vi "Send Command.vi"(8 "error in (no error)":errorcluster, 10 "Command":u8(ring)=27 items=["Cancel"=24, "Clear"=25, "CSR"=28, "Echo"=27, "Filter"=15, "Gcal"=18, "Goto"=16, "Grtid?"=19, "Grtsel"=26, "NOVRAM Read"=56, "NOVRAM Write"=59, "Reset"=255, "Scan"=12, "Scan Up"=9, "Scan Down"=3, "Serial?"=33, "Slew Up"=8, "Slew Down"=2, "Slit Reset"=43, "Slit?"=30, "Sltadj"=14, "Speed"=13, "Speed?"=21, "Step Down"=1, "Step Up"=7, "S1adj"=31, "S2adj"=32, "S3adj"=34, "S1cal"=22, "S2cal"=23, "S3cal"=35, "Test"=17, "Type"=57, "Wave?"=29, "Zero"=52], 11 "VISA resource name":refnum<visa-resource-name>) -> (0 "error out":errorcluster, 2 "response":u8, 3 "VISA resource name out":refnum<visa-resource-name>)   [LabVIEW 2012, in "Digikrom DK24x.lvlib"]
doc: "Begins the communication sequence for the specified command."
uses:
  Digikrom DK24x.lvlib
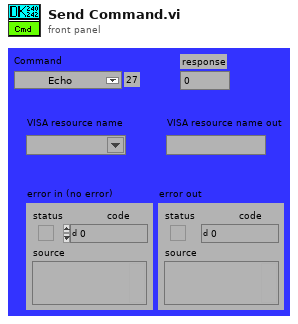
[diagram p1: front panel]
types:
  T1 = typedef "Semaphore RefNum" = refnum<k1>
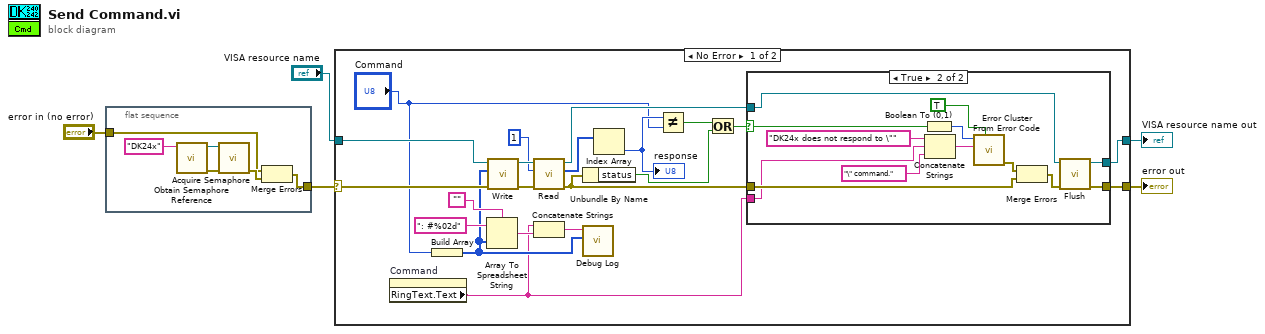
[diagram p0: block diagram]
diagram:
  n1 = flat-sequence {
    tunnel: "error in (no error)" -> [w7]
    tunnel: [w6] -> w1
    frame #0 {
      n2 = call <vilib>:"Obtain Semaphore Reference.vi"("name (unnamed)"="DK24x") -> ("error out"=w9:errorcluster, "semaphore"=w10:T1)  [unwired: 2 in, 3 out]
      n3 = call <vilib>:"Acquire Semaphore.vi"("error in (no error)"=w9, "semaphore"=w10) -> ("error out"=w8:errorcluster)  [unwired: 1 in, 4 out]
      n4 = Merge Errors(w7, w8) -> (w6:errorcluster)
    }
  }
  n5 = case shown="No Error" w1 {
    selector: w1 -> [w19 w48]
    tunnel: "VISA resource name" -> [w32 w49]
    tunnel: [w27 w48] -> w4
    tunnel: [w24 w49] -> w3
    frame No Error {
      n6 = property on="Command" class="Ring (strict)"() -> ("RingText.Text"=w12:string)  [unwired: 2 in, 2 out]
      n7 = Build Array("Command") -> (w14:u8[])
      n8 = Array To Spreadsheet String(delimiter (Tab)="", array=w14, 3:": #%02d" ("format string")) -> (spreadsheet string=w16:string)
      n9 = call "Write.vi"("error in (no error)"=w19, "Byte Array"=w14, "VISA resource name"=w32) -> ("error out"=w29:errorcluster, "VISA resource name out"=w30:refnum<visa-resource-name>)  [unwired: 7 out]
      n10 = call "Read.vi"("error in (no error)"=w29, "response size"=1, "VISA resource name"=w30) -> ("error out"=w23:errorcluster, "response array"=w31:u8[], "VISA resource name out"=w25:refnum<visa-resource-name>)  [unwired: 6 out]
      n11 = Concatenate Strings(w12, w16) -> (w15:string)
      n12 = Unbundle By Name(w23) -> ("status"=w20:bool)
      n13 = call "Debug Log.vi"("Data"=w14, "Message"=w15) -> ()  [unwired: 2 in, 8 out]
      n14 = Index Array(array=w31) -> (element=w26:u8)  [unwired: 1 in]
      "response" <- w26
      n15 = Not Equal?(x=w26, y="Command") -> (x != y?=w21:bool)
      n16 = Or(x=w21, y=w20) -> (x .or. y?=w22:bool)
      n17 = case shown="True" w22 {
        selector: w22 -> [_ w39]
        tunnel: w23 -> [w34 w42]
        tunnel: [w34 w45] -> w27
        tunnel: w25 -> [w33 w47]
        tunnel: [w33 w46] -> w24
        tunnel: w12 -> [_ w36]
        frame False {
        }
        frame True {
          n18 = Boolean To (0,1)(Boolean=w39) -> (0, 1=w38:i16)
          n19 = Concatenate Strings("DK24x does not respond to \"", w36, "\" command." ("string")) -> (w37:string)
          n20 = call <vilib>:"Error Cluster From Error Code.vi"("show call chain? (False)"=TRUE, "error message (\"\")"=w37, "error code (0)"=w38) -> ("error out"=w41:errorcluster)  [unwired: 1 in, 5 out]
          n21 = Merge Errors(w41, w42) -> (w40:errorcluster)
          n22 = call "Flush.vi"("error in (no error)"=w40, "VISA resource name"=w47) -> ("error out"=w45:errorcluster, "VISA resource name out"=w46:refnum<visa-resource-name>)  [unwired: 8 out]
        }
      }
    }
    frame Error {
    }
  }
  "error out" <- w4
  "VISA resource name out" <- w3
